vi "VPA QC View Notes.vi"(8 "error in (no error)":errorcluster, 10 "State Cluster in":T1) -> (0 "error out":errorcluster, 2 "State Cluster out":T1)   [LabVIEW 2013]
uses:
  Controls/VPA QC State Data Cluster.ctl
  Controls/VPA QC General Cluster.ctl
  Controls/VPA QC State Enum.ctl
  Controls/VPA QC Bool Cluster.ctl
panel:
  in  "Ok":bool
  in  "Delete":bool
  in  "Add Comment":bool
  in  "Notes":i32(listbox)
  # "Assembly Checklist"
  # "Assembly Checklist"
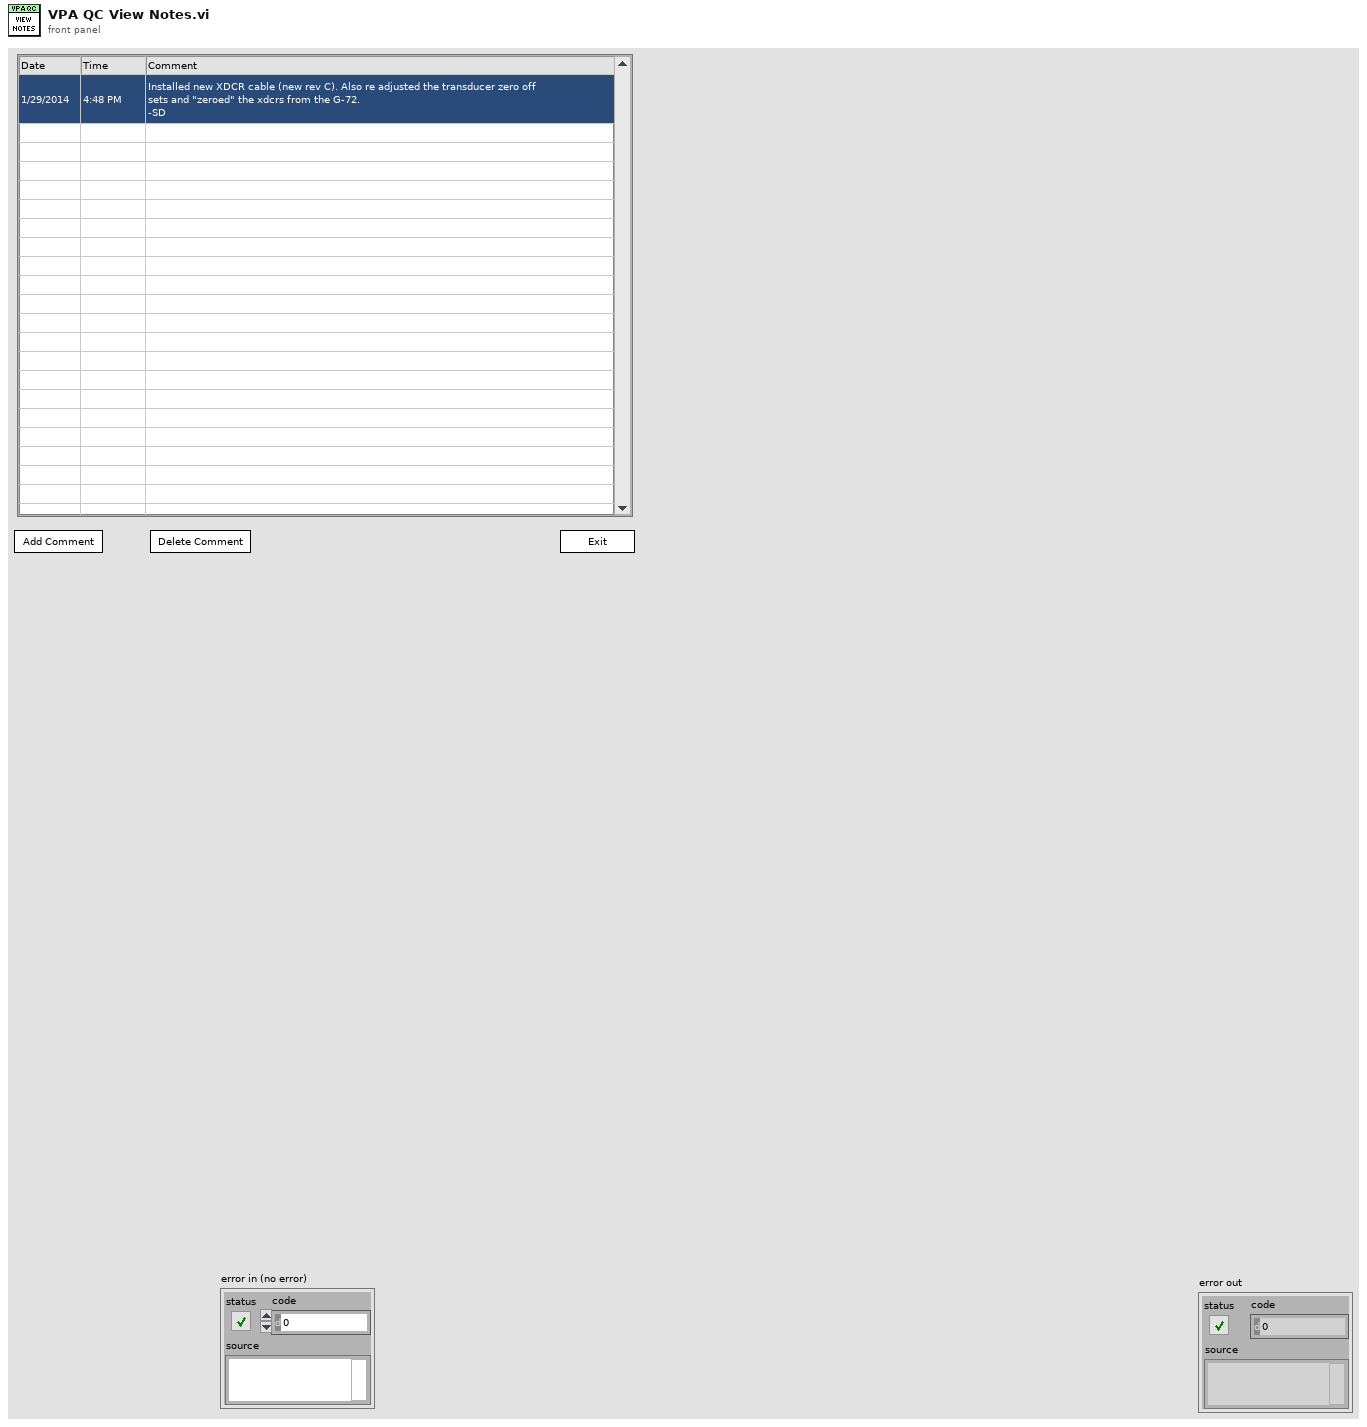
[diagram p1: front panel]
types:
  T1 = typedef "VPA QC State Data Cluster.ctl" = cluster{"XDCR 1":tag, "XDCR 2":tag, "General Information Clust":T2, "Assembly Checklist":cluster{"Ensure Drive Assembly checklist is completed.":bool, "Tighten Screws":bool, "Ensure VPA is wired correctly.":bool, "Ensure pump is running at voltage specified by customer.":bool}, "State":T3, "Manifold Leak Test Data":dbl[][], "Pressure Verification Test Data":dbl[][], "Flow Mode Verification Data":dbl[][], "DAQmx Error":errorcluster, "Bool Cluster":T4, "Leak Test Start Time":timestamp, "Pressure Test Start Time":timestamp, "Flow Test Start Time":timestamp, "Final Checklist cluster":cluster{"Check Fact Rest":bool, "Initialize Pump":bool, "Maintenance Hours":bool, "Clean Water Out":bool, "Covers":bool, "Screws":bool, "Wrap":bool, "Box":bool, "Clear Error Log":bool}, "Volts Constant":dbl, "Volume Constant A":dbl, "Volume Constant B":dbl, "Save File Path":path, "Comments Array":string[][], "File Format Version":u16}
  T2 = typedef "VPA QC General Cluster.ctl" = cluster{"Tech Name":string, "Date":timestamp, "Customer":string, "VPA Model":string, "G-72 Software Version":string, "Galil SN":string, "Galil Software Version":string, "VPA SN":string, "Valve SN":string, "Side A Drive Module SN":string, "Side B Drive Module SN":string, "A Side Transducer SN":string, "B Side Transducer SN":string, "A Side Motor SN":string, "B Side Motor SN":string, "A Side Gear Reducer SN":string, "B Side Gear Reducer SN":string, "A Side Limit Switch SN":string, "B Side Limit Switch SN":string, "Pump Voltage":string}
  T3 = typedef "VPA QC State Enum.ctl" = enum16{"General Information", "XDCR and LS Check", "Check Pump Function", "Manifold/Cylinder Leak Test", "Exit"}
  T4 = typedef "VPA QC Bool Cluster.ctl" = cluster{"Assembly":bool, "Gen":bool, "XDCR and LS Setup":bool, "Verify Pump Operation":bool, "Leak Test":bool, "Calibrate XDCRs":bool, "P Mode Verify":bool, "F Mode Verify":bool, "Vol Calibration":bool, "Flow Rate Test":bool, "Final Checklist":bool}
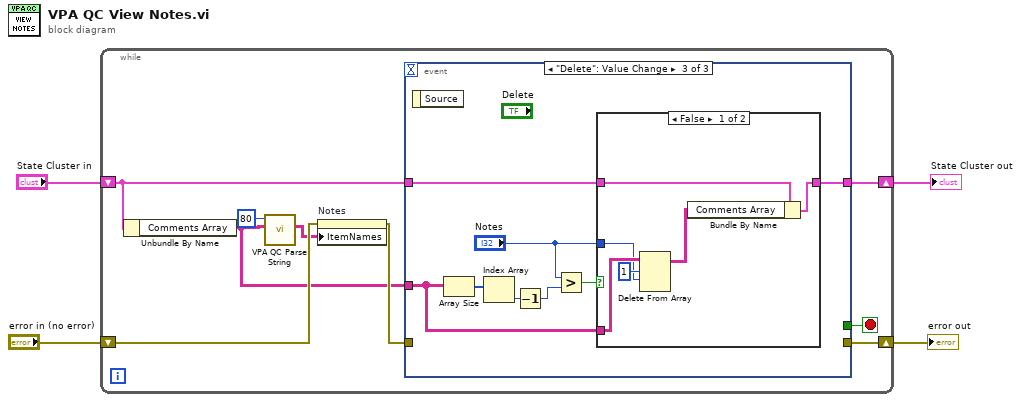
[diagram p0: block diagram]
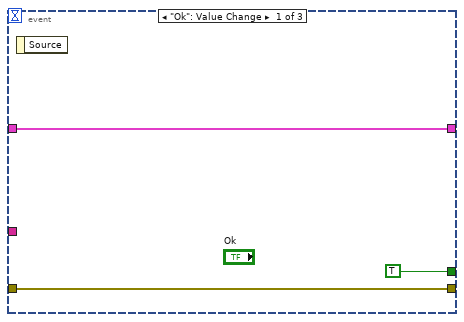
[diagram p2: hidden frame]
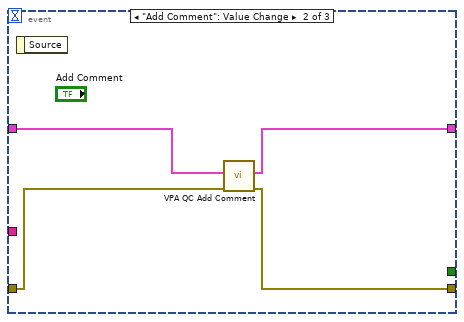
[diagram p3: hidden frame]
diagram:
  n1 = while {
    shift-right: [w12] -> w4
    shift-left: "error in (no error)" -> [w9]
    shift-right: [w11] -> w3
    shift-left: "State Cluster in" -> [w8]
    stop <- w13 stop-if-true
    n2 = Unbundle By Name(w8) -> ("Comments Array"=w6:string[][])
    n3 = call "VPA QC Parse String.vi"("Strings In"=w6, "Max Line Length"=80) -> ("Strings Out"=w5:string[][])  [unwired: 9 in]
    n4 = property on="Notes" class="MCListbox (strict)"(error in=w9, "ItemNames"=w5) -> (error out=w10:errorcluster)  [unwired: 1 in, 1 out]
    n5 = event shown="[2] \"Delete\": Value Change" {
      selector: _ -> [_ _ _]
      dyn-events: _ -> [_ _ _]
      timeout: _ -> [_ _ _]
      tunnel: [TRUE _ _] -> w13
      tunnel: w10 -> [w15 w18 _]
      tunnel: [w15 w17 _] -> w12
      tunnel: w8 -> [w14 w20 w22]
      tunnel: [w14 w19 w21] -> w11
      tunnel: w6 -> [_ _ w23]
      event "Ok": Value Change {
        n6 = event-data() -> ()  [unwired: 1 in, 1 out]
      }
      event "Add Comment": Value Change {
        n7 = event-data() -> ()  [unwired: 1 in, 1 out]
        n8 = call "VPA QC Add Comment.vi"("error in (no error)"=w18, "State Cluster In"=w20) -> ("error out"=w17:errorcluster, "State Cluster Out"=w19:T1)  [unwired: 8 in]
      }
      event "Delete": Value Change {
        n9 = event-data() -> ()  [unwired: 1 in, 1 out]
        n10 = Array Size(array=w23) -> (size(s)=w28:i32[])
        n11 = Index Array(array=w28) -> (element=w27:i32)  [unwired: 1 in]
        n12 = Decrement(x=w27) -> (x-1=w26:i32)
        n13 = Greater?(x="Notes", y=w26) -> (0:w25:bool)
        n14 = case shown="False" w25 {
          tunnel: "Notes" -> [w32 _]
          tunnel: w23 -> [w34 _]
          tunnel: w22 -> [w31 w35]
          tunnel: [w29 w35] -> w21
          frame False {
            n15 = Delete From Array(array=w34, length=1, index (row)=w32) -> (array with subset deleted=w30:string[][])  [unwired: 1 in, 1 out]
            n16 = Bundle By Name(cluster=w31, "Comments Array"=w30) -> (w29:T1)
          }
          frame True {
            # "Null Entry Selected"
          }
        }
      }
    }
  }
  "State Cluster out" <- w3
  "error out" <- w4
